vi "Main.vi"() -> ()   [LabVIEW 2014]
uses:
  Normal Proxy Pattern/Proxy/OperationLogger (proxy).lvclass
panel:
  in  "Enum":enum16{"Subject 1", "Subject 2"}(ring)=enum."Subject 2"
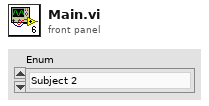
[diagram p1: front panel]
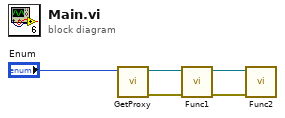
[diagram p0: block diagram]
diagram:
  n1 = call "GetProxy.vi"("Enum"="Enum") -> ("error out"=w2:errorcluster, "OperationLogger (proxy) out"=w3:refnum<class "OperationLogger (proxy).lvclass">)  [unwired: 9 in]
  n2 = call-dynamic "Func1.vi"("error in (no error)"=w2, "OperationLogger (proxy) in"=w3) -> ("error out"=w4:errorcluster, "OperationLogger (proxy) out"=w5:refnum<class "OperationLogger (proxy).lvclass">)  [unwired: 8 in]
  n3 = call-dynamic "Func2.vi"("error in (no error)"=w4, "OperationLogger (proxy) in"=w5) -> ()  [unwired: 8 in, 2 out]
